vi "Execute Eulogy.vi"(6 "Mouse Position":T1, 8 "User VI Ref":refnum<vi>, 9 "Menu Item Tag Suffix":string, 10 "Remaining Items":refnum<vi>[](array[refnum]), 11 "Affected Items":T2) -> (0 "Fail transaction?":bool)   [LabVIEW 2017, in "Shortcut Menu.lvlib"]
doc: "This VI is part of a plug-in for modifying the LabVIEW shortcut menus. This is the execute VI which is called when the shortcut menu is chosen by the user. It performs the action of the selected menu item."
uses:
  Shortcut Menu.lvlib
  Eulogy.ctl
  <vilib>/Utility/miscctls.llb/LVPositionTypeDef.ctl
  Toolkit VIs/Toolkit VIs.lvlib
panel:
  # "All controls on this panel except \"Affected Items\" have been locked to prevent accidental edits. Changing the control names or types, other than the elements of the \"Affected Items\" cluster will make the VI unusable as a menu plugin.\n\nSee Context Help for each control for details about its use."
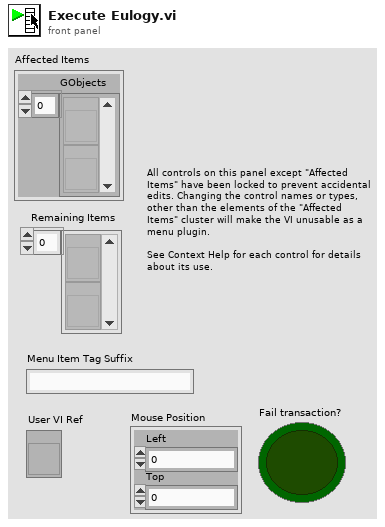
[diagram p1: front panel]
types:
  T1 = typedef "LVPositionTypeDef.ctl" = cluster{"Left":i32, "Top":i32}
  T2 = typedef "Shortcut Menu.lvlib/Eulogy.ctl" = cluster{"GObjects":refnum<vi>[]}
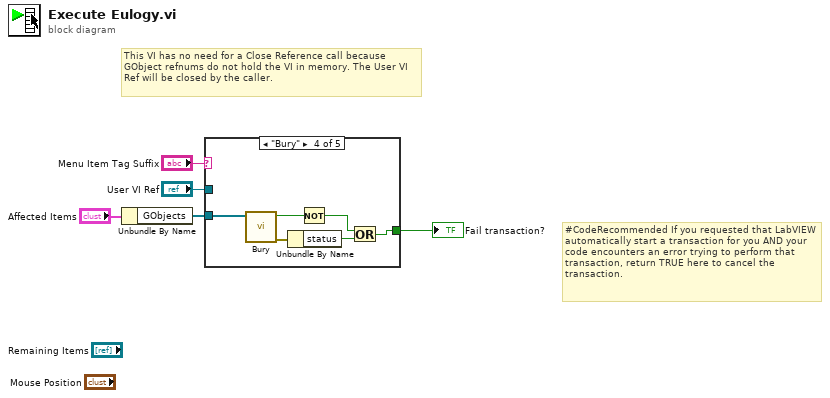
[diagram p0: block diagram]
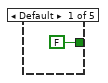
[diagram p2: hidden frame]
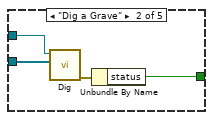
[diagram p3: hidden frame]
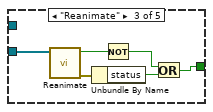
[diagram p4: hidden frame]
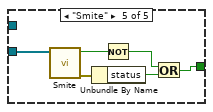
[diagram p5: hidden frame]
diagram:
  # "#CodeRecommended If you requested that LabVIEW automatically start a transaction for you AND your code encounters an error trying to perform that transaction, return TRUE here to cancel the transaction."
  # "This VI has no need for a Close Reference call because GObject refnums do not hold the VI in memory. The User VI Ref will be closed by the caller."
  n1 = Unbundle By Name("Affected Items") -> ("GObjects"=w2:refnum<vi>[])
  n2 = case shown="\"Bury\"" "Menu Item Tag Suffix" {
    tunnel: [FALSE ("Fail transaction?") w7 w11 w18 w23] -> w3
    tunnel: w2 -> [_ w10 w12 w17 w24]
    tunnel: "User VI Ref" -> [_ w9 _ _ _]
    frame Default {
    }
    frame "Dig a Grave" {
      n3 = call "Dig.vi"("Selection List[]"=w10, "VI In"=w9) -> ("Error Out"=w8:errorcluster)  [unwired: 8 in, 1 out]
      n4 = Unbundle By Name(w8) -> ("status"=w7:bool)
    }
    frame "Reanimate" {
      n5 = call "Reanimate.vi"("Selection List[]"=w12) -> ("Error Out"=w14:errorcluster, "Change Made?"=w16:bool)  [unwired: 9 in]
      n6 = Unbundle By Name(w14) -> ("status"=w13:bool)
      n7 = Not(x=w16) -> (.not. x?=w15:bool)
      n8 = Or(x=w15, y=w13) -> (x .or. y?=w11:bool)
    }
    frame "Bury" {
      n9 = call "Bury.vi"("Selection List[]"=w17) -> ("Error Out"=w20:errorcluster, "Change Made?"=w22:bool)  [unwired: 9 in]
      n10 = Unbundle By Name(w20) -> ("status"=w19:bool)
      n11 = Not(x=w22) -> (.not. x?=w21:bool)
      n12 = Or(x=w21, y=w19) -> (x .or. y?=w18:bool)
    }
    frame "Smite" {
      n13 = call "Smite.vi"("Selection List[]"=w24) -> ("Error Out"=w26:errorcluster, "Change Made?"=w28:bool)  [unwired: 9 in]
      n14 = Unbundle By Name(w26) -> ("status"=w25:bool)
      n15 = Not(x=w28) -> (.not. x?=w27:bool)
      n16 = Or(x=w27, y=w25) -> (x .or. y?=w23:bool)
    }
  }
  "Fail transaction?" <- w3
